vi "LauncherAngleTalon.vi"() -> ()   [LabVIEW 2012]
uses:
  State_Machine_Enum.ctl
  RefnameEnum.ctl
  Robot Global Data.vi
panel:
  in  "Start at bottom?":bool=TRUE
  in  "LSBackwardValue":dbl=-0.7999999999999999 min=-1.0 max=0.0 step=0.1
  in  "LSForwardValue":dbl=0.7999999999999999 min=0.0 max=1.0 step=0.1
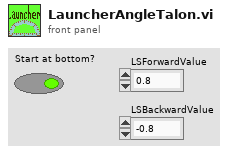
[diagram p1: front panel]
types:
  T1 = typedef "State_Machine_Enum.ctl" = enum16{"Idle", "Start", "Do", "Stop", "Init"}
  T2 = typedef "RefnameEnum.ctl" = enum16{"FireLauncher", "Climber", "Shield", "TankDrive", "DriveEncoderL", "DriveEncoderR", "LauncherMotorRPM", "LauncherEncoderAnalog", "LauncherEncoderRPM", "ShooterLS", "DriveAlignLS", "ClimbingLS", "LauncherEncoderAngle", "LauncherMotorAngle", "Gamepad1", "Gamepad2", "Compressor"}
  T3 = typedef "LoopDisable.ctl" = cluster{"Climb.vi":bool, "LauncherAngle.vi":bool, "Launcher.vi":bool, "ArmControl.vi":bool, "WinchMotor.vi":bool, "ReadDriveEncoder.vi":bool}
  T4 = typedef "WPI_DigitalInputDevRef.ctl" = cluster{"DevStatus":errorcluster, "DIO Channel":T5, "Digital Module":T6}
  T5 = typedef "FPGA_DIOChannel.ctl" = enum8{"DIO 1", "DIO 2", "DIO 3", "DIO 4", "DIO 5", "DIO 6", "DIO 7", "DIO 8", "DIO 9", "DIO 10", "DIO 11", "DIO 12", "DIO 13", "DIO 14", "Invalid"}
  T6 = typedef "FPGA_TypedefDigitalModule.ctl" = enum16{"Digital Module 1", "Digital Module 2"}
  T7 = typedef "WPI_EncoderDevRef.ctl" = cluster{"DevStatus":errorcluster, "EncoderIndex":T8, "CounterIndex":T9, "DistancePerCount":dbl, "Decoding Type":T10}
  T8 = typedef "FPGA_EncoderIdx.ctl" = enum8{"Enc 0", "Enc 1", "Enc 2", "Enc 3", "Invalid"}
  T9 = typedef "FPGA_CounterCtrSystemIndex.ctl" = enum8{"Ctr 0", "Ctr 1", "Ctr 2", "Ctr 3", "Ctr 4", "Ctr 5", "Ctr 6", "Ctr 7", "Invalid"}
  T10 = typedef "WPI_EncoderType.ctl" = enum16{"1x", "2x", "4x"}
  T11 = typedef "WPI_MotorControlDeviceRef.ctl" = cluster{"DeviceStatus":errorcluster, "Type":enum16{"PWM", "CAN"}, "PWM":cluster{"Digital Module":T6, "PWM Channel":T12, "DeadBand":T13}, "CAN":cluster{"Device Number":u8, "Control Mode":T14, "Semaphore":T15, "Max Vout":dbl}, "Invert":bool, "TransformRef":T16, "InvTransformRef":T16}
  T12 = typedef "FPGA_DIOPWMChannel.ctl" = enum8{"PWM 1", "PWM 2", "PWM 3", "PWM 4", "PWM 5", "PWM 6", "PWM 7", "PWM 8", "PWM 9", "PWM 10", "Invalid"}
  T13 = typedef "WPI_PWMDeadband.ctl" = cluster{"Name":string, "maxPositivePwm":i32, "minPositivePwm":i32, "centerPwm":i32, "maxNegativePwm":i32, "minNegativePwm":i32, "angularRange":u16}
  T14 = typedef "WPI_CANJaguar_ControlMode.ctl" = enum8{"Percent VBus", "Current", "Speed", "Position", "Voltage"}
  T15 = typedef "Semaphore RefNum" = refnum<k1>
  T16 = typedef "WPI_PWMTransform_ConPane.ctl" = refnum<vi>
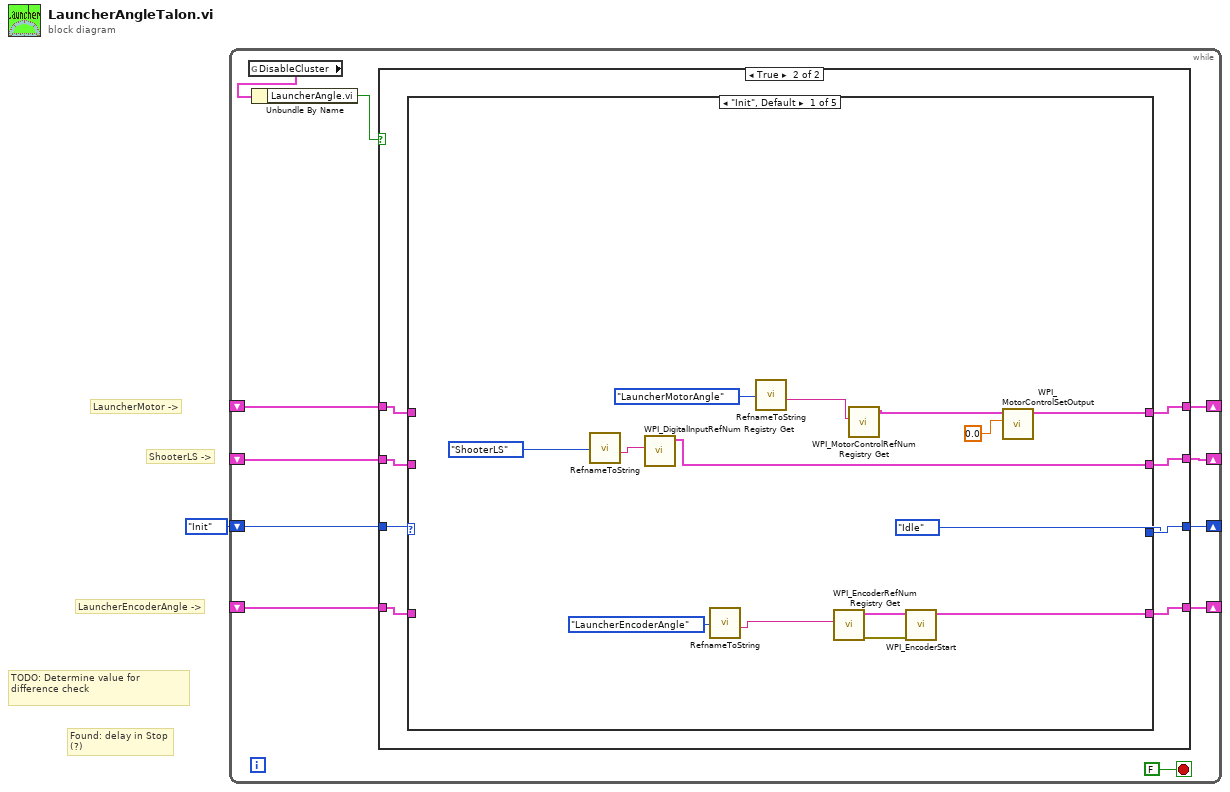
[diagram p0: block diagram]
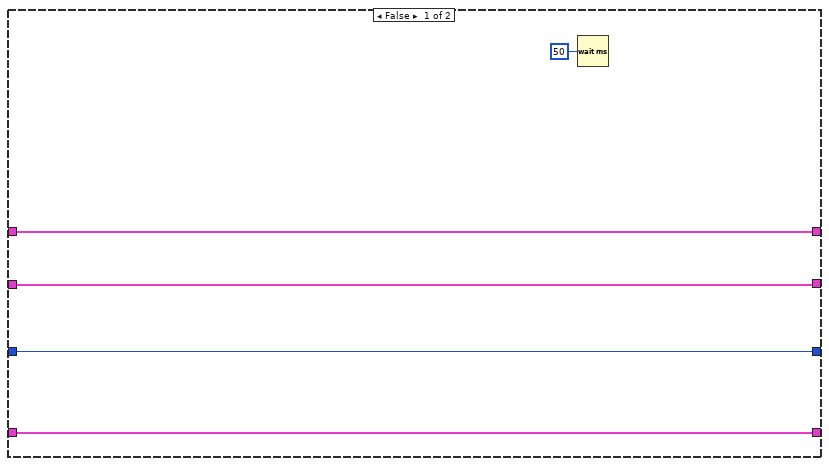
[diagram p2: hidden frame]
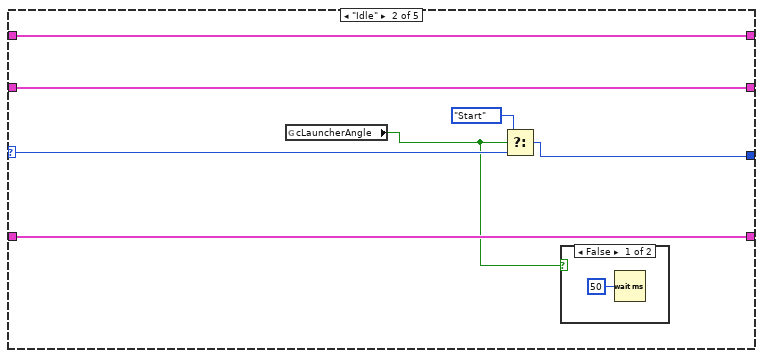
[diagram p3: hidden frame]
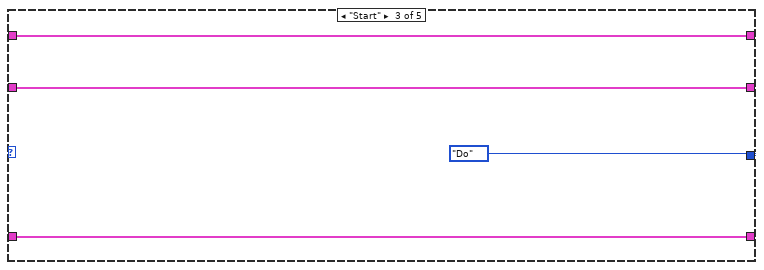
[diagram p5: hidden frame]
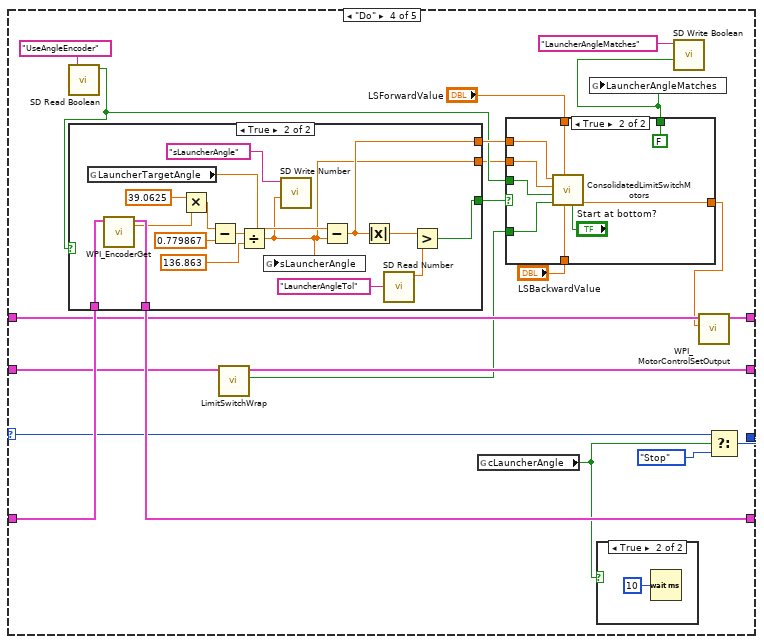
[diagram p6: hidden frame]
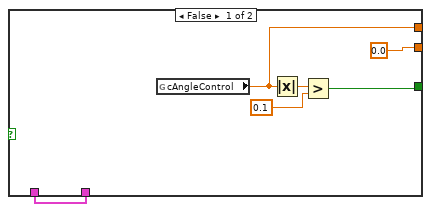
[diagram p7: hidden frame]
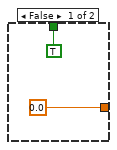
[diagram p9: hidden frame]
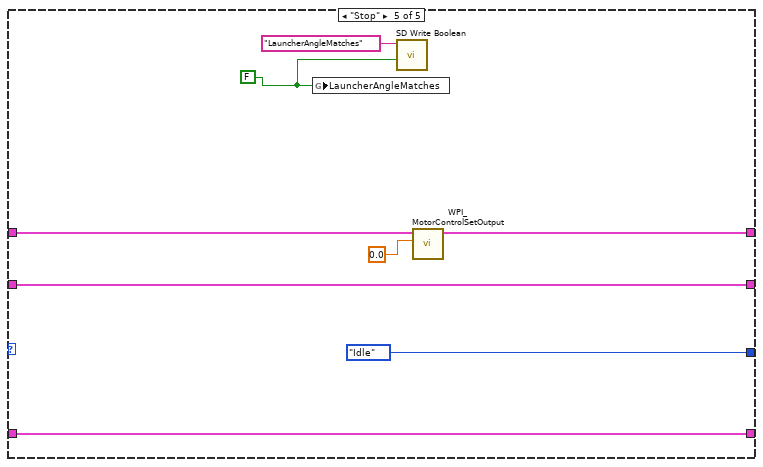
[diagram p10: hidden frame]
diagram:
  # "ShooterLS ->"
  # "Found: delay in Stop \n(?)"
  # "TODO: Determine value for difference check"
  # "LauncherEncoderAngle ->"
  # "LauncherMotor ->"
  n1 = while {
    shift-right: [w10] -> _
    shift-left: State_Machine_Enum."Init" ("State") -> [w11]
    shift-right: [w9] -> _
    shift-left: _ -> [w8]
    shift-right: [w4] -> _
    shift-left: _ -> [w3]
    shift-right: [w6] -> _
    shift-left: _ -> [w7]
    stop <- FALSE stop-if-true
    n2 = global read "Robot Global Data.vi" "DisableCluster"() -> (w5:T3)
    n3 = Unbundle By Name(w5) -> ("LauncherAngle.vi"=w2:bool)
    n4 = case shown="True" w2 {
      tunnel: w11 -> [w16 w25]
      tunnel: [w16 w24] -> w10
      tunnel: [w15 w23] -> w9
      tunnel: w8 -> [w15 w22]
      tunnel: w7 -> [w17 w21]
      tunnel: [w17 w20] -> w6
      tunnel: [w13 w19] -> w4
      tunnel: w3 -> [w13 w18]
      frame False {
        n5 = Wait (ms)(milliseconds to wait=u32 50) -> ()  [unwired: 1 out]
      }
      frame True {
        n6 = case shown="\"Init\", Default" w25 {
          selector: w25 -> [_ w44 _ w69 _]
          tunnel: [State_Machine_Enum."Idle" ("State") w45 State_Machine_Enum."Do" ("State") w68 State_Machine_Enum."Idle" ("State")] -> w24
          tunnel: [w37 w42 w50 w70 w114] -> w23
          tunnel: w22 -> [_ w42 w50 w71 w114]
          tunnel: w21 -> [_ w43 w49 w58 w113]
          tunnel: [w35 w43 w49 w57 w113] -> w20
          tunnel: [w34 w40 w48 w63 w111] -> w19
          tunnel: w18 -> [_ w40 w48 w64 w112]
          frame "Init", Default {
            n7 = call "RefnameToString.vi"("Enum"=RefnameEnum."ShooterLS") -> ("Refname"=w28:string)  [unwired: 10 in]
            n8 = call <vilib>:"WPI_DigitalInputRefNum Registry Get.vi"("refnum name"=w28) -> ("DigitalInputDevRef"=w35:T4)  [unwired: 9 in, 1 out]
            n9 = call "RefnameToString.vi"("Enum"=RefnameEnum."LauncherEncoderAngle") -> ("Refname"=w26:string)  [unwired: 10 in]
            n10 = call "RefnameToString.vi"("Enum"=RefnameEnum."LauncherMotorAngle") -> ("Refname"=w30:string)  [unwired: 10 in]
            n11 = call <vilib>:"WPI_EncoderRefNum Registry Get.vi"("refnum name"=w26) -> ("error out"=w36:errorcluster, "EncoderDevRef"=w38:T7)  [unwired: 9 in]
            n12 = call <vilib>:"WPI_MotorControlRefNum Registry Get.vi"("refnum name"=w30) -> ("MotorControlDevRef"=w32:T11)  [unwired: 9 in, 1 out]
            n13 = call <vilib>:"WPI_EncoderStart.vi"("error in (no error)"=w36, "EncoderDevRef"=w38) -> ("EncoderDevRef"=w37:T7)  [unwired: 8 in, 1 out]
            n14 = call <vilib>:"WPI_MotorControlSetOutput.vi"("Output"=0.0, "MotorControlDevRef"=w32) -> ("MotorControlDevRef"=w34:T11)  [unwired: 7 in, 2 out]
          }
          frame "Idle" {
            n15 = global read "Robot Global Data.vi" "cLauncherAngle"() -> (w41:bool)
            n16 = Select(t=State_Machine_Enum."Start" ("State"), s=w41, f=w44) -> (s? t:f=w45:T1)
            n17 = case shown="False" w41 {
              frame False {
                n18 = Wait (ms)(milliseconds to wait=u32 50) -> ()  [unwired: 1 out]
              }
              frame True {
              }
            }
          }
          frame "Start" {
          }
          frame "Do" {
            n19 = call <vilib>:"SD Read Boolean.vi"("Name"="UseAngleEncoder") -> ("Boolean"=w53:bool)  [unwired: 8 in, 2 out]
            n20 = case shown="True" w53 {
              tunnel: w71 -> [w74 w94]
              tunnel: [w74 w93] -> w70
              tunnel: [w75 w91] -> w67
              tunnel: [w76 w90] -> w66
              tunnel: [0.0 w81] -> w52
              frame False {
                n21 = global read "Robot Global Data.vi" "cAngleControl"() -> (w75:dbl)
                n22 = Absolute Value(x=w75) -> (abs(x)=w78:dbl)
                n23 = Greater?(x=w78, y=0.1) -> (0:w76:bool)
              }
              frame True {
                n24 = global read "Robot Global Data.vi" "LauncherTargetAngle"() -> (w86:dbl)
                n25 = call <vilib>:"WPI_EncoderGet.vi"("EncoderDevRef"=w94) -> ("Distance"=w83:dbl, "EncoderDevRef"=w93:T7)  [unwired: 5 in, 4 out]
                n26 = Multiply(x=39.0625, y=w83) -> (x*y=w82:dbl)
                n27 = Subtract(x=w82, y=0.779867) -> (x-y=w89:dbl)
                n28 = Divide(x=w89, y=136.863) -> (x/y=w81:dbl)
                n29 = global write "Robot Global Data.vi" "sLauncherAngle"(w81) -> ()
                n30 = call <vilib>:"SD Write Number.vi"("Numeric"=w81, "Name"="sLauncherAngle") -> ()  [unwired: 8 in, 2 out]
                n31 = Subtract(x=w86, y=w81) -> (x-y=w91:dbl)
                n32 = Absolute Value(x=w91) -> (abs(x)=w92:dbl)
                n33 = call <vilib>:"SD Read Number.vi"("Name"="LauncherAngleTol") -> ("Numeric"=w79:dbl)  [unwired: 8 in, 2 out]
                n34 = Greater?(x=w92, y=w79) -> (0:w90:bool)
              }
            }
            n35 = call "LimitSwitchWrap.vi"("DigitalInputDevRef"=w58) -> ("Triggered"=w56:bool, "DigitalInputDevRef 2"=w57:T4)  [unwired: 9 in]
            n36 = global read "Robot Global Data.vi" "cLauncherAngle"() -> (w65:bool)
            n37 = case shown="True" w66 {
              tunnel: w67 -> [_ w102]
              tunnel: [0.0 ("New Output") w106] -> w60
              tunnel: w56 -> [_ w105]
              tunnel: "LSBackwardValue" -> [_ w104]
              tunnel: "LSForwardValue" -> [_ w103]
              tunnel: [TRUE FALSE] -> w54
              tunnel: w53 -> [_ w98]
              tunnel: w52 -> [_ w99]
              frame False {
              }
              frame True {
                n38 = call "ConsolidatedLimitSwitchMotors.vi"("Start at bottom?"="Start at bottom?", "BackwardValue"=w104, "ForwardValue"=w103, "CurrentLSValue"=w105, "UsingEncoder?"=w98, "AngleEncoderValue"=w99, "CurrentInput"=w102) -> ("New Output"=w106:dbl)  [unwired: 4 in]
              }
            }
            n39 = global write "Robot Global Data.vi" "LauncherAngleMatches"(w54) -> ()
            n40 = case shown="True" w65 {
              frame False {
              }
              frame True {
                n41 = Wait (ms)(milliseconds to wait=u32 10) -> ()  [unwired: 1 out]
              }
            }
            n42 = call <vilib>:"SD Write Boolean.vi"("Boolean"=w54, "Name"="LauncherAngleMatches") -> ()  [unwired: 8 in, 2 out]
            n43 = call <vilib>:"WPI_MotorControlSetOutput.vi"("Output"=w60, "MotorControlDevRef"=w64) -> ("MotorControlDevRef"=w63:T11)  [unwired: 7 in, 2 out]
            n44 = Select(t=w69, s=w65, f=State_Machine_Enum."Stop" ("State")) -> (s? t:f=w68:T1)
          }
          frame "Stop" {
            w107 = FALSE
            n45 = global write "Robot Global Data.vi" "LauncherAngleMatches"(w107) -> ()
            n46 = call <vilib>:"SD Write Boolean.vi"("Boolean"=w107, "Name"="LauncherAngleMatches") -> ()  [unwired: 8 in, 2 out]
            n47 = call <vilib>:"WPI_MotorControlSetOutput.vi"("Output"=0.0, "MotorControlDevRef"=w112) -> ("MotorControlDevRef"=w111:T11)  [unwired: 7 in, 2 out]
          }
        }
      }
    }
  }
